vi "PowerEnergyMeter_param.vi"() -> ()   [LabVIEW 2018]
panel:
  in  "能量计量程":enum16{"200uJ", "20uJ", "2uJ", "200nJ"}(ring)
  in  "能量计通道":enum16{"Channel 1", "Channel 2"}(ring)=enum."Channel 2"
  in  "功率计通道":enum16{"Channel 1", "Channel 2"}(ring)
  in  "测量表头IP":string="192.168.129.20"
  # "能量功率计\n参数"
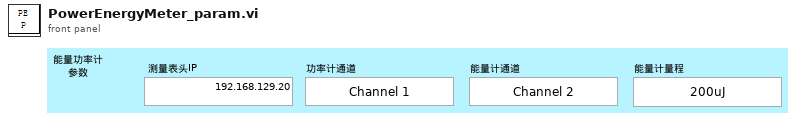
[diagram p1: front panel]
types:
  T1 = typedef "IMAQ Image.ctl" = refnum<image>
  T2 = cluster{"示波器":cluster{"Channel (0:Channel 1)":enum16{"Channel 1", "Channel 2", "Channel 3", "Channel 4"}, "电压范围":dbl, "触发电压":dbl, "时间范围":dbl, " 示波器VISA":refnum<visa-resource-name>, "时间范围 标签":u64, "电压范围 标签":u64, "触发电压 标签":u64, "输入阻抗/Ω":u64, "示波器类型":bool}, "光谱仪":cluster{"SpecDataReference":refnum<queue>, "grating center":dbl, "Exposure Time (s)":dbl, "是否进行详细设置":bool, " 开始通信检查":bool, "通信成功？":bool, "波长":dbl, "LightField Automation out":refnum<class "LightField Automation.lvclass">}, " 近场相机":cluster{"曝光时间/us":dbl, "IP 地址":string, "ImageData":T1, " 曝光最大":i32, " 曝光最小":i32, "Camera Source":refnum<k21>, "近场X范围":dbl, "近场Y范围":dbl, "单个像元大小/um":dbl, "相机距离原点位置":dbl[], "是否测量发散角":bool, "光束类型(发散T)":bool, "聚焦透镜焦距mm":dbl}, " 偏振仪":cluster{"电压范围":u64, "触发电压":u64, "时间范围":u64, "波长范围":enum16{"可见光 400-700nm", "近红外 700-1100nm"}, "可见光偏振测量仪VISA":refnum<visa-resource-name>, "近红外偏振测量仪VISA":refnum<visa-resource-name>}, " 功率计":cluster{"通道":enum16{"Channel 1", "Channel 2"}, "工作波长":u32, "单位":u64, "时间范围":u64, "IP地址":string, "端口":u32, "是否需要散射片":bool}, "能量计":cluster{"通道":enum16{"Channel 1", "Channel 2"}, "工作波长":u32, "单位":u64, "时间范围":u64, "IP地址":string, "端口":u32, "能量计量程":enum16{"200uJ", "20uJ", "2uJ", "200nJ"}}, "电机":cluster{"Channel (0:Channel 1)":enum16{"Channel 1", "Channel 2", "Channel 3", "Channel 4"}, "电压范围":u64, "触发电压":u64, "时间范围":u64}, " 远场相机":cluster{"曝光时间":i32, "IP 地址":string, "ImageData":T1, "  增益最大":i32, "  增益最小":i32, " 曝光最大":i32, " 曝光最小":i32, "ImageData B":T1, "是否远场测量":bool}}
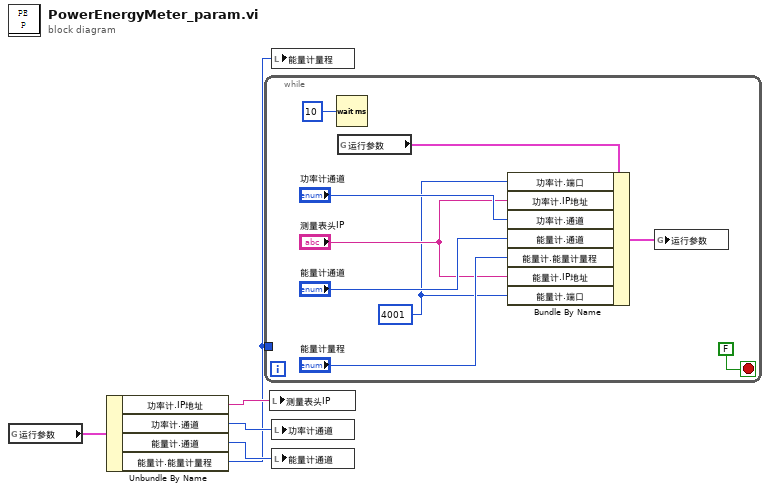
[diagram p0: block diagram]
diagram:
  n1 = global read "参数.vi" "运行参数"() -> (w5:T2)
  n2 = Unbundle By Name(w5) -> ("功率计.IP地址"=w3:string, "功率计.通道"=w4:enum16{"Channel 1", "Channel 2"}, "能量计.通道"=w2:enum16{"Channel 1", "Channel 2"}, "能量计.能量计量程"=w1:enum16{"200uJ", "20uJ", "2uJ", "200nJ"})
  n3 = while {
    tunnel: w1 -> [_]
    stop <- FALSE stop-if-true
    w6 = u32 4001 ("能量计.端口")
    n4 = Wait (ms)(milliseconds to wait=u32 10 ("等待时间（毫秒）")) -> ()  [unwired: 1 out]
    n5 = global read "参数.vi" "运行参数"() -> (w12:T2)
    n6 = Bundle By Name(cluster=w12, "功率计.端口"=w6, "功率计.IP地址"="测量表头IP", "功率计.通道"="功率计通道", "能量计.通道"="能量计通道", "能量计.能量计量程"="能量计量程", "能量计.IP地址"="测量表头IP", "能量计.端口"=w6) -> (w11:T2)
    n7 = global write "参数.vi" "运行参数"(w11) -> ()
  }
  n8 = local write "测量表头IP"(w3) -> ()
  n9 = local write "能量计量程"(w1) -> ()
  n10 = local write "功率计通道"(w4) -> ()
  n11 = local write "能量计通道"(w2) -> ()
